vi "Close.vi"(8 "error in":errorcluster, 11 "Chiller Cluster - 1 Channel.lvclass":refnum<class "Power Supply Cluster - 1 Channel.lvclass">) -> (0 "error out":errorcluster)   [LabVIEW 2023, in "Power Supply Cluster - 1 Channel.lvclass"]
uses:
  Power Supply Cluster - 1 Channel.lvclass
  Power Supply Cluster - 1 Channel.lvclass/Power Supply Cluster - 1 Channel.ctl
  <vilib>/ADAS Replay HIL/AdasHilServices/AdasHilServices Fill In Error Info Ex.vi
  <vilib>/ADAS Replay HIL/AdasHilServices/AdasHilChannelServices.lvlib
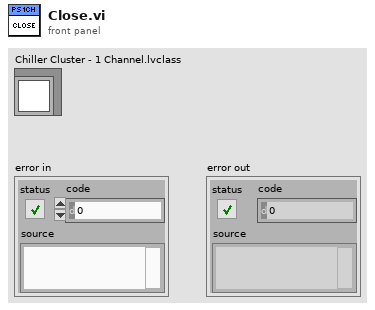
[diagram p1: front panel]
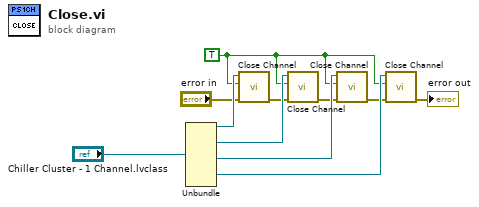
[diagram p0: block diagram]
diagram:
  w4 = TRUE ("Force Destroy? (F)")
  n1 = Unbundle("Chiller Cluster - 1 Channel.lvclass") -> (w10:refnum<k21>, w9:refnum<k21>, w6:refnum<k21>, w5:refnum<k21>)  [unwired: 4 out]
  n2 = call <vilib>:"Close Channel.vi"("error in"="error in", "Force Destroy? (F)"=w4, "ADAS HIL Channel"=w10) -> ("error out"=w7:errorcluster)  [unwired: 8 in]
  n3 = call <vilib>:"Close Channel.vi"("error in"=w7, "Force Destroy? (F)"=w4, "ADAS HIL Channel"=w9) -> ("error out"=w3:errorcluster)  [unwired: 8 in]
  n4 = call <vilib>:"Close Channel.vi"("error in"=w3, "Force Destroy? (F)"=w4, "ADAS HIL Channel"=w6) -> ("error out"=w2:errorcluster)  [unwired: 8 in]
  n5 = call <vilib>:"Close Channel.vi"("error in"=w2, "Force Destroy? (F)"=w4, "ADAS HIL Channel"=w5) -> ("error out"=→"error out":errorcluster)  [unwired: 8 in]
